vi "ReadWriteGlobalPreferences.vi"(7 "Task":enum16{"Read", "Save", "Clear"}(ring), 9 "Last Test":string, 10 "plots":refnum<vi>[](array[refnum])) -> (2 "Last Test Out":string)   [LabVIEW 2024]
uses:
  <vilib>/Utility/miscctls.llb/LVRangeTypeDef.ctl
panel:
  in  "Default":T2={"X Range"=[{"Minimum"=200.0, "Maximum"=10000.0, "Increment"=2500.0, "Minor Increment"=500.0, "Start"=2500.0}, {"Minimum"=0.0, "Maximum"=0.05, "Increment"=0.025, "Minor Increment"=0.0025, "Start"=0.0}, {"Minimum"=0.0, "Maximum"=0.3, "Increment"=0.1, "Minor Increment"=0.01, "Start"=0.0}, {"Minimum"=200.0, "Maximum"=10000.0, "Increment"=10.0, "Minor Increment"=100.0, "Start"=1000.0}], "Y Range"=[{"Minimum"=-25.0, "Maximum"=0.0, "Increment"=5.0, "Minor Increment"=1.0, "Start"=-25.0}, {"Minimum"=-100.0, "Maximum"=100.0, "Increment"=50.0, "Minor Increment"=10.0, "Start"=-100.0}, {"Minimum"=-100.0, "Maximum"=100.0, "Increment"=50.0, "Minor Increment"=10.0, "Start"=-100.0}, {"Minimum"=-30.0, "Maximum"=30.0, "Increment"=5.0, "Minor Increment"=1.0, "Start"=-30.0}], "Last Test"="ScratchPad"}
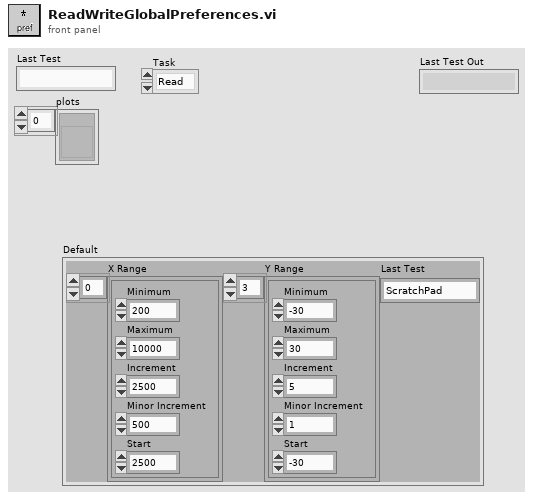
[diagram p1: front panel]
types:
  T1 = typedef "LVRangeTypeDef.ctl" = cluster{"Minimum":dbl, "Maximum":dbl, "Increment":dbl, "Minor Increment":dbl, "Start":dbl}
  T2 = cluster{"X Range":T1[], "Y Range":T1[], "Last Test":string}
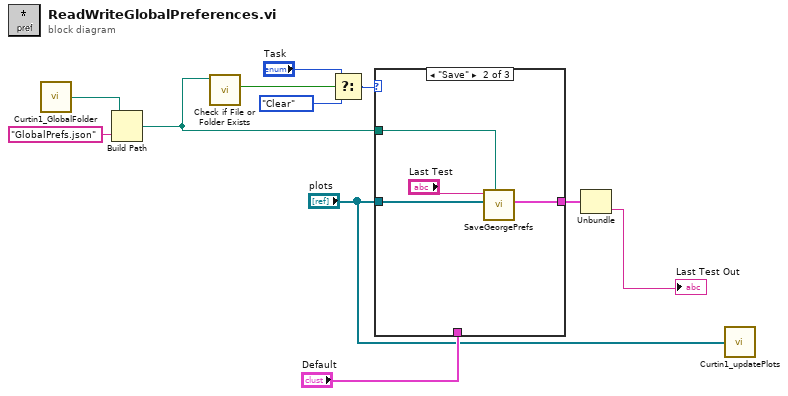
[diagram p0: block diagram]
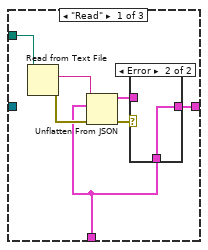
[diagram p2: hidden frame]
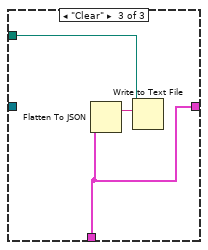
[diagram p4: hidden frame]
diagram:
  n1 = call "Curtin1_GlobalFolder.vi"() -> ("LabVIEW Data Path"=w2:path)  [unwired: 1 in]
  n2 = Build Path(base path=w2, name or relative path="GlobalPrefs.json") -> (appended path=w4:path)
  n3 = call <vilib>:"Check if File or Folder Exists.vi"("path"=w4) -> ("file or folder exists?"=w10:bool)  [unwired: 8 in, 2 out]
  n4 = Select(t="Task", s=w10, f=enum16{"Read", "Save", "Clear"}."Clear") -> (s? t:f=w8:enum16{"Read", "Save", "Clear"})
  n5 = case shown="\"Save\"" w8 {
    tunnel: w4 -> [w18 w21 w27]
    tunnel: [w14 w22 w25] -> w1
    tunnel: "Default" -> [w12 _ w25]
    tunnel: "plots" -> [_ w23 _]
    frame "Read" {
      n6 = Read from Text File(file (use dialog)=w18) -> (text=w17:string, error out=w16:errorcluster)  [unwired: 3 in, 2 out]
      n7 = Unflatten From JSON(JSON string=w17, type and defaults=w12, error in (no error)=w16) -> (value=w13:T2, error out=w15:errorcluster)  [unwired: 4 in]
      n8 = case shown="Error" w15 {
        tunnel: [w19 w20] -> w14
        tunnel: w13 -> [w19 _]
        tunnel: w12 -> [_ w20]
        frame No Error {
        }
        frame Error {
        }
      }
    }
    frame "Save" {
      n9 = call "SaveGeorgePrefs.vi"("GlobalPrefs"=w21, "plots"=w23, "Test Name"="Last Test") -> ("Settings"=w22:T2)  [unwired: 7 in, 1 out]
    }
    frame "Clear" {
      n10 = Flatten To JSON(anything=w25) -> (JSON string=w26:string)  [unwired: 2 in, 1 out]
      n11 = Write to Text File(file (use dialog)=w27, text=w26) -> ()  [unwired: 2 in, 3 out]
    }
  }
  n12 = Unbundle(w1) -> ("Last Test"=→"Last Test Out":string)  [unwired: 2 out]
  n13 = call "Curtin1_updatePlots.vi"("plots"="plots") -> ()  [unwired: 11 in]
